vi "setting cable.vi"(8 "error in (no error)":errorcluster, 11 "시험 모드":T1) -> (0 "error out":errorcluster)   [LabVIEW 2019]
uses:
  Test Mode.ctl
panel:
  out "String":string
  in  "Exit":bool
  in  "Tab Control":enum32{"저전압모드 동작", "접촉저항", "고전압모드 동작"}(tab)
  # "케이블 & 전류 프로브 설정"
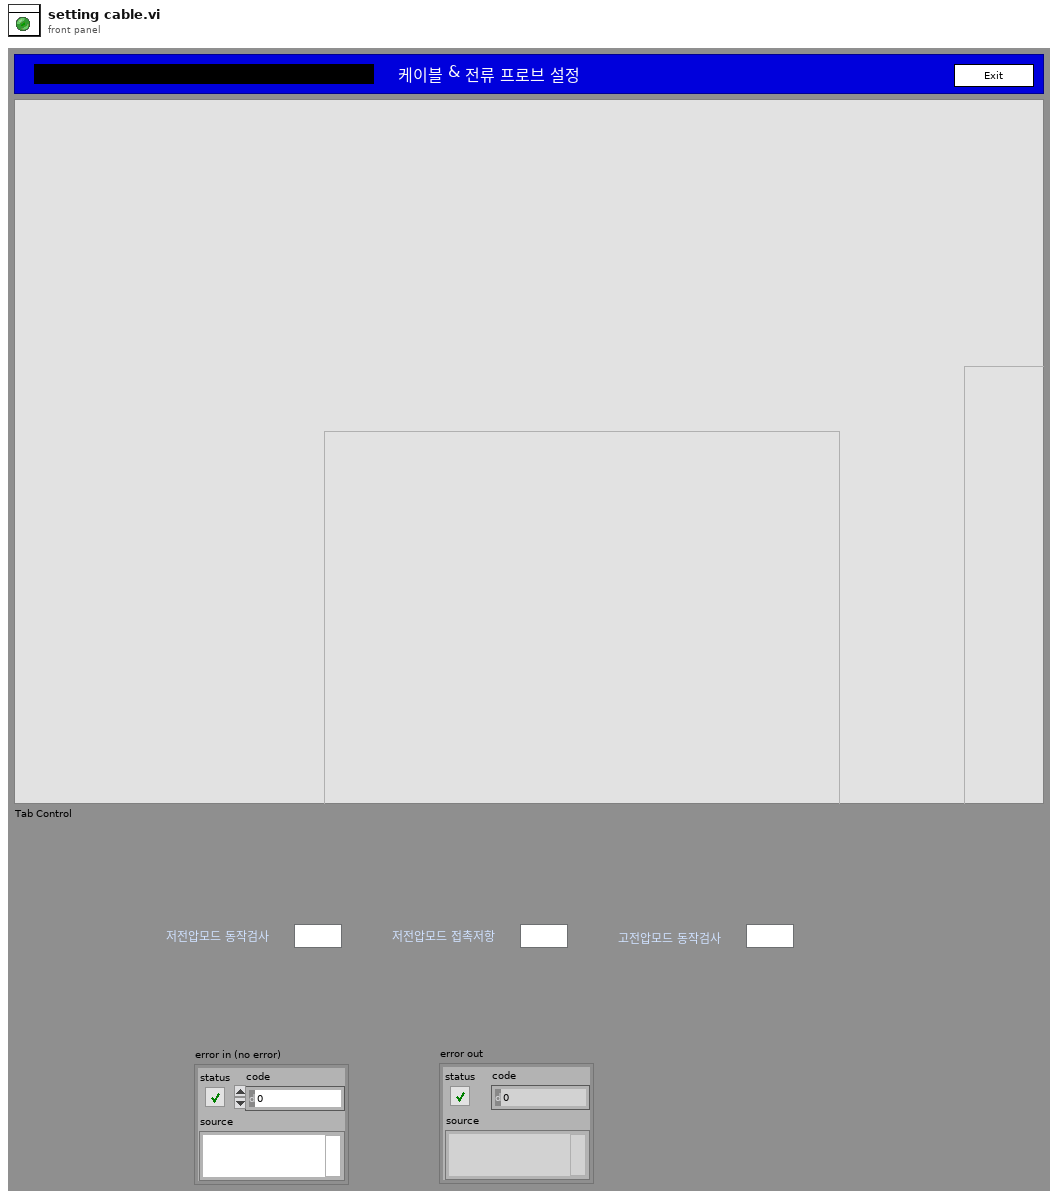
[diagram p1: front panel]
types:
  T1 = typedef "Test Mode.ctl" = enum32{"저항부하", "캐패시터부하", "B수명 - 1", "B수명 - 2", "B수명 - 3", "저전압모드 동작검사", "저전압모드 접촉저항", "고전압모드 동작검사"}
  T2 = enum32{"Invalid", "Standard", "Closed", "Hidden", "Minimized", "Maximized"}
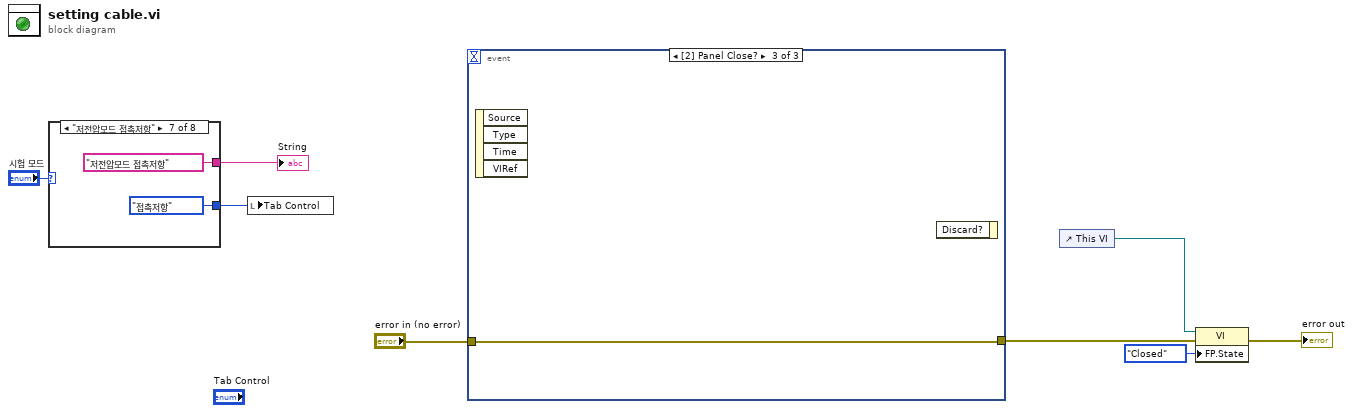
[diagram p0: block diagram]
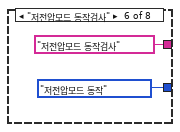
[diagram p7: hidden frame]
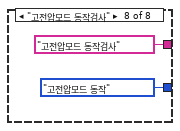
[diagram p8: hidden frame]
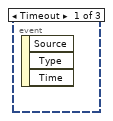
[diagram p9: hidden frame]
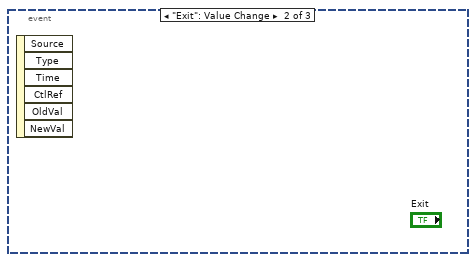
[diagram p10: hidden frame]
diagram:
  n1 = case shown="\"저전압모드 접촉저항\"" "시험 모드" {
    tunnel: [_ _ _ _ _ enum32{"저전압모드 동작", "접촉저항", "고전압모드 동작"}."저전압모드 동작" ("Tab Control") enum32{"저전압모드 동작", "접촉저항", "고전압모드 동작"}."접촉저항" ("Tab Control") enum32{"저전압모드 동작", "접촉저항", "고전압모드 동작"}."고전압모드 동작" ("Tab Control")] -> w2
    tunnel: [_ _ _ _ _ "저전압모드 동작검사" ("String") "저전압모드 접촉저항" ("String") "고전압모드 동작검사" ("String")] -> w1
    frame "저항부하", Default {
    }
    frame "캐패시터부하" {
    }
    frame "B수명 - 1" {
    }
    frame "B수명 - 2" {
    }
    frame "B수명 - 3" {
    }
    frame "저전압모드 동작검사" {
    }
    frame "저전압모드 접촉저항" {
    }
    frame "고전압모드 동작검사" {
    }
  }
  "String" <- w1
  n2 = local write "Tab Control"(w2) -> ()
  n3 = event shown="[2] Panel Close?" {
    selector: _ -> [_ _ _]
    dyn-events: _ -> [_ _ _]
    timeout: _ -> [_ _ _]
    tunnel: [_ _ w15] -> w7
    tunnel: "error in (no error)" -> [_ _ w15]
    event Timeout {
      n4 = event-data() -> ()  [unwired: 1 in, 3 out]
    }
    event "Exit": Value Change {
      n5 = event-data() -> ()  [unwired: 1 in, 6 out]
    }
    event Panel Close? {
      n6 = event-data() -> ()  [unwired: 1 in, 4 out]
      n7 = event-data() -> ()  [unwired: 2 in, 1 out]
    }
  }
  n8 = control-ref of="This VI"() -> (w6:refnum<vi>)
  n9 = property class="VI"(reference=w6, error in=w7, "FP.State"=T2."Closed" ("Front Panel Window:State")) -> (error out=→"error out":errorcluster)  [unwired: 1 out]
